vi "Show UI.vi"(0 "reference in":refnum<class "User Manager.lvclass">, 2 "UI Type":T1, 5 "Error In":errorcluster) -> (14 "reference out":refnum<class "User Manager.lvclass">, 19 "Error Out":errorcluster)   [LabVIEW 2024, in "User Manager.lvclass"]
uses:
  User Manager.lvclass
  UIType.ctl
  User Manager.lvclass/User Manager.ctl
panel:
  # "Connector Pane"
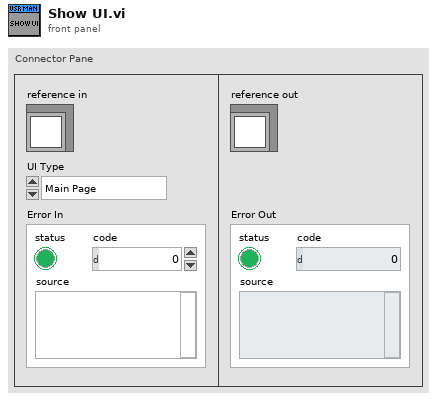
[diagram p1: front panel]
types:
  T1 = typedef "UIType.ctl" = enum16{"Main Page", "Settings Page", "Debugging Page"}
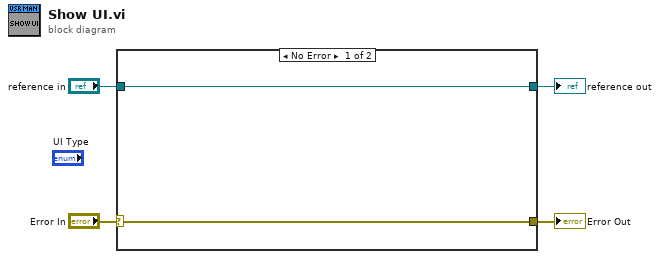
[diagram p0: block diagram]
diagram:
  n1 = case shown="No Error" "Error In" {
    selector: "Error In" -> [w5 w8]
    tunnel: [w5 w8] -> w3
    tunnel: [w6 w7] -> w1
    tunnel: "reference in" -> [w6 w7]
    frame No Error {
    }
    frame Error {
    }
  }
  "Error Out" <- w3
  "reference out" <- w1
